vi "flush_syringe.vi"(6 "Flush Volume (mL)":dbl=1.0 min=0.0 max=2.5 step=0.1, 8 "Syringe Flushes":i32=3, 9 "Sample Port":u16(ring) items=["A"=1, "B"=2, "C"=3, "D"=4, "E"=5, "F"=6, "G"=7, "H"=8], 10 "kloehn session in":T1={"VISA resource out"="COM12", "error out"={"status"=FALSE, "code"=0, "source"=""}}, 11 "relay session in":T1={"VISA resource out"="COM12", "error out"={"status"=FALSE, "code"=0, "source"=""}}) -> (2 "kloehn session out":T1={"VISA resource out"="COM12", "error out"={"status"=FALSE, "code"=0, "source"=""}}, 3 "relay session out":T1={"VISA resource out"="COM12", "error out"={"status"=FALSE, "code"=0, "source"=""}})   [LabVIEW 2010]
panel:
  # "Later, this VI should be rewritten in order to make selection of a new port quicker (by knowing whether clockwise or counter clockwise is going to be fastest)."
  # "This VI leaves the syring on port A and will expect the get_sample VI to switch the syringe to the sample port. Sample port is still needed here though for pullin in the sample that nees to be flushed through the system."
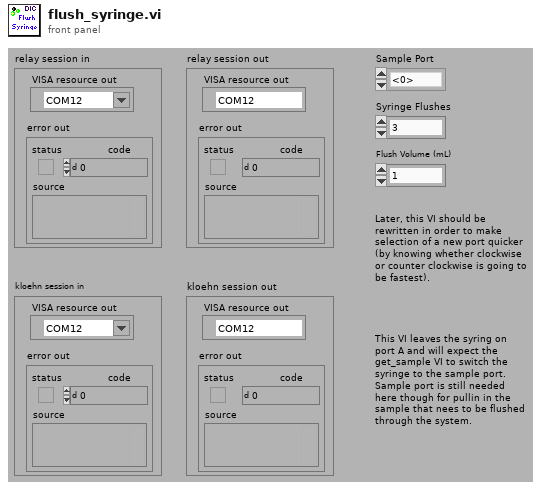
[diagram p1: front panel]
types:
  T1 = cluster{"VISA resource out":refnum<visa-resource-name>, "error out":errorcluster}
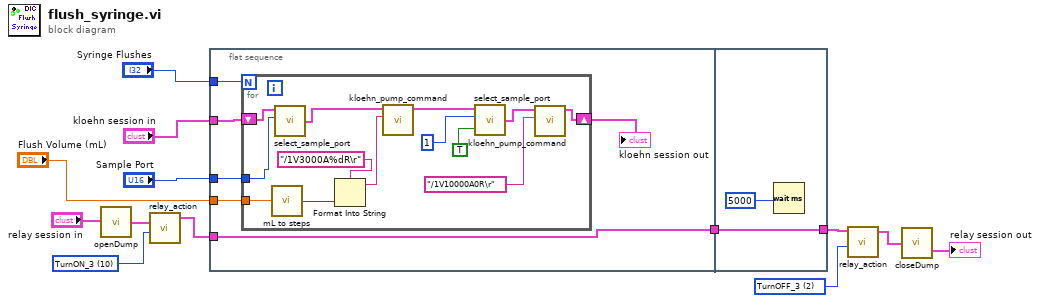
[diagram p0: block diagram]
diagram:
  w2 = u8 2 items=["OPEN DUMP ON_1"=8, "TurnON_PUMP"=9, "TurnON_3"=10, "TurnON_4"=11, "CLOSE DUMP OFF_1"=0, "TurnOFF_PUMP"=1, "TurnOFF_3"=2, "TurnOFF_4"=3, "OpenAll"=30, "CloseAllRelay"=29] ("Action")
  w9 = u8 10 items=["OPEN DUMP ON_1"=8, "TurnON_PUMP"=9, "TurnON_3"=10, "TurnON_4"=11, "CLOSE DUMP OFF_1"=0, "TurnOFF_PUMP"=1, "TurnOFF_3"=2, "TurnOFF_4"=3, "OpenAll"=30, "CloseAllRelay"=29] ("Action")
  n1 = call "openDump.vi"("relay session in"="relay session in") -> ("relay session out"=w8:T1)
  n2 = call "relay_action.vi"("relay session in"=w8, "Action"=w9) -> ("relay session out"=w6:T1)  [unwired: 6 in]
  n3 = flat-sequence {
    tunnel: "Syringe Flushes" -> [w18]
    tunnel: "kloehn session in" -> [w17]
    tunnel: "Sample Port" -> [w16]
    tunnel: [w15] -> w7
    tunnel: w6 -> [w15]
    tunnel: "Flush Volume (mL)" -> [w14]
    tunnel: w7 -> [w34]
    tunnel: [w34] -> w5
    frame #0 {
      n4 = for {
        N: w18 -> [_]
        shift-right: [w29] -> w19
        shift-left: w17 -> [w31]
        tunnel: w16 -> [w30]
        tunnel: w14 -> [w21]
        n5 = call "mL to steps.vi"("mL in"=w21) -> ("steps out"=w20:i32)
        n6 = call "select_sample_port.vi"("Sample Port"=w30, "kloehn session in"=w31) -> ("kloehn session out"=w26:T1)  [unwired: 2 in]
        n7 = Format Into String(format string="/1V3000A%dR\r", w20) -> (resulting string=w22:string)  [unwired: 2 in, 1 out]
        n8 = call "kloehn_pump_command.vi"("Send String"=w22, "kloehn session in"=w26) -> ("kloehn session out"=w25:T1)  [unwired: 6 in, 3 out]
        n9 = call "select_sample_port.vi"("counter-clockwise?"=TRUE, "Sample Port"=1, "kloehn session in"=w25) -> ("kloehn session out"=w24:T1)  [unwired: 1 in]
        n10 = call "kloehn_pump_command.vi"("Send String"="/1V10000A0R\r", "kloehn session in"=w24) -> ("kloehn session out"=w29:T1)  [unwired: 6 in, 3 out]
      }
      "kloehn session out" <- w19
    }
    frame #1 {
      n11 = Wait (ms)(milliseconds to wait=5000) -> ()  [unwired: 1 out]
    }
  }
  n12 = call "relay_action.vi"("relay session in"=w5, "Action"=w2) -> ("relay session out"=w3:T1)  [unwired: 6 in]
  n13 = call "closeDump.vi"("relay session in"=w3) -> ("relay session out"=→"relay session out":T1)
